vi "Machine - Add Device (SubVI).vi"(8 "error in":errorcluster, 10 "IP Address/SN":string[](array[string]), 11 "Port":string[](array[string])) -> (0 "error out":errorcluster)   [LabVIEW 2019]
uses:
  Controls/Machine - Device Type.ctl
  Controls/Sensor Setup - State.ctl
  Controls/Sensor Setup - Data Structure.ctl
  Controls/Calibration - Data Structure.ctl
  Controls/eFGV States.ctl
  Controls/Global - Data UDP.vi
panel:
  in  "Device Type":T1 items=["Unitron", "Flowtron", "Datalogger"]
  in  "Port":string
  in  "IP Address/SN List":i32(listbox)
  in  "IP Address/SN":string
  in  "Device Name":string
  in  "Status":u16(ring) items=["ACTIVE", "DISABLE"]
  in  "Close":bool
  in  "Save":bool
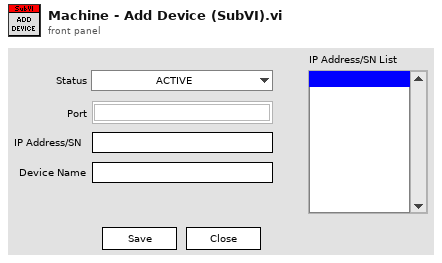
[diagram p1: front panel]
types:
  T1 = typedef "Machine - Device Type.ctl" = u16
  T2 = typedef "Sensor Setup - State.ctl" = enum16{"Init", "Idle", "Save", "Close"}
  T3 = typedef "Sensor Setup - Data Structure.ctl" = cluster{"serialno":string, "Name":string, "Channel":string, "Slope":string, "Intercept":string, "Unit":string, "Decimal":string, "New?":bool, "Data":T4, "Port":string[], "IP/SN":string[]}
  T4 = typedef "Calibration - Data Structure.ctl" = cluster{"Timeout":i32, "LC MC":dbl[], "TD MC":dbl[], "Motor Pulse":u64, "Disp M":dbl[], "LC Unit":string[], "Disp Unit":string[], "TD Unit":string[], "LC Name":string[], "TD Name":string[], "Machine":enum16{"Please Select", "Motor 1", "Motor 2", "Motor 3", "Motor 4", "Motor 5", "Motor 6", "Motor 7", "Motor 8", "Motor 9"}, "Sensor Port":enum16{"Please Select", "LC 1", "LC 2", "LC 3", "LC 4", "LC 5", "LC 6", "LC 7", "LC 8", "TD 1", "TD 2", "TD 3", "TD 4", "TD 5", "TD 6", "TD 7", "TD 8", "TD 9", "TD 10", "TD 11", "TD 12"}[]}
  T5 = typedef "eFGV States.ctl" = enum16{"Init", "Read", "Write", "Exit"}
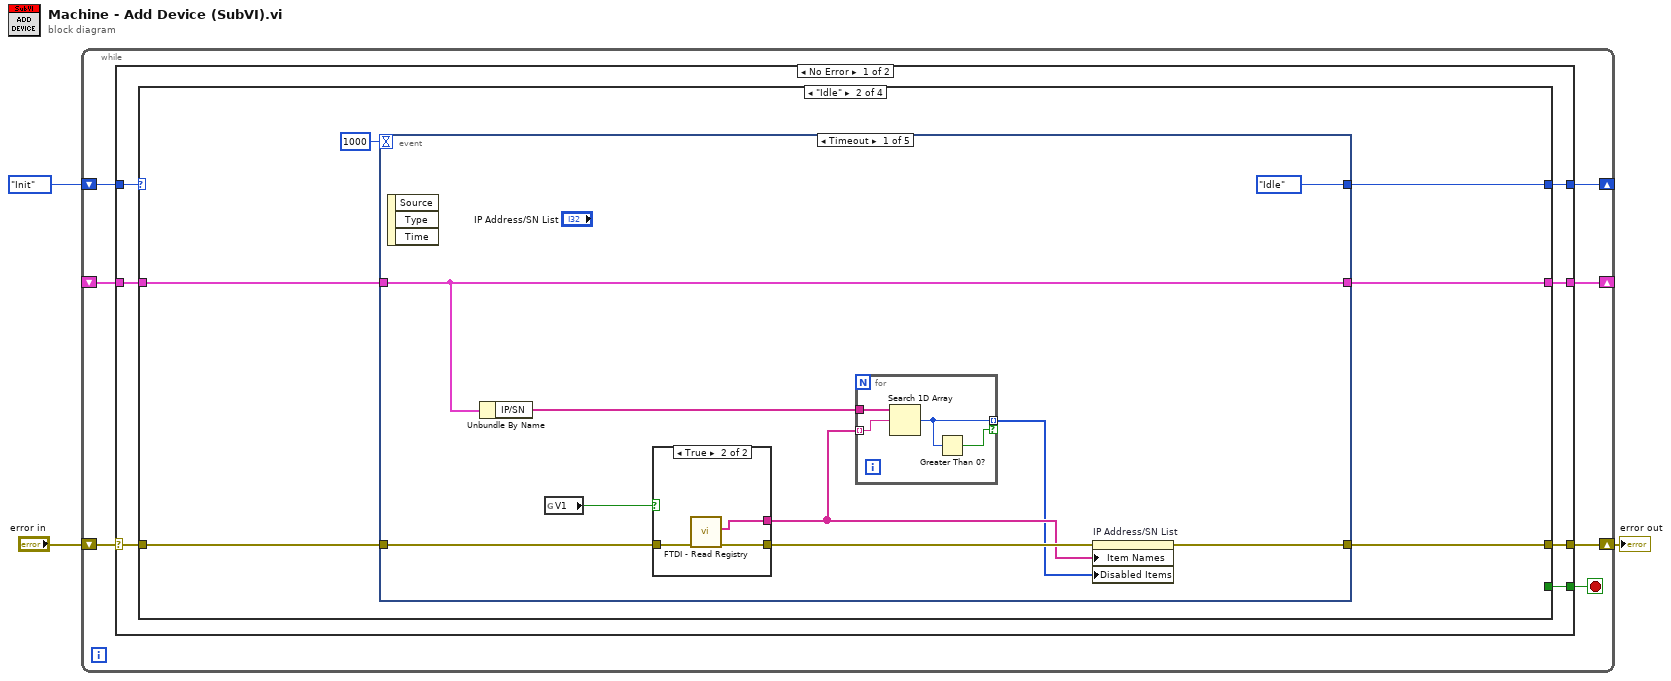
[diagram p0: block diagram]
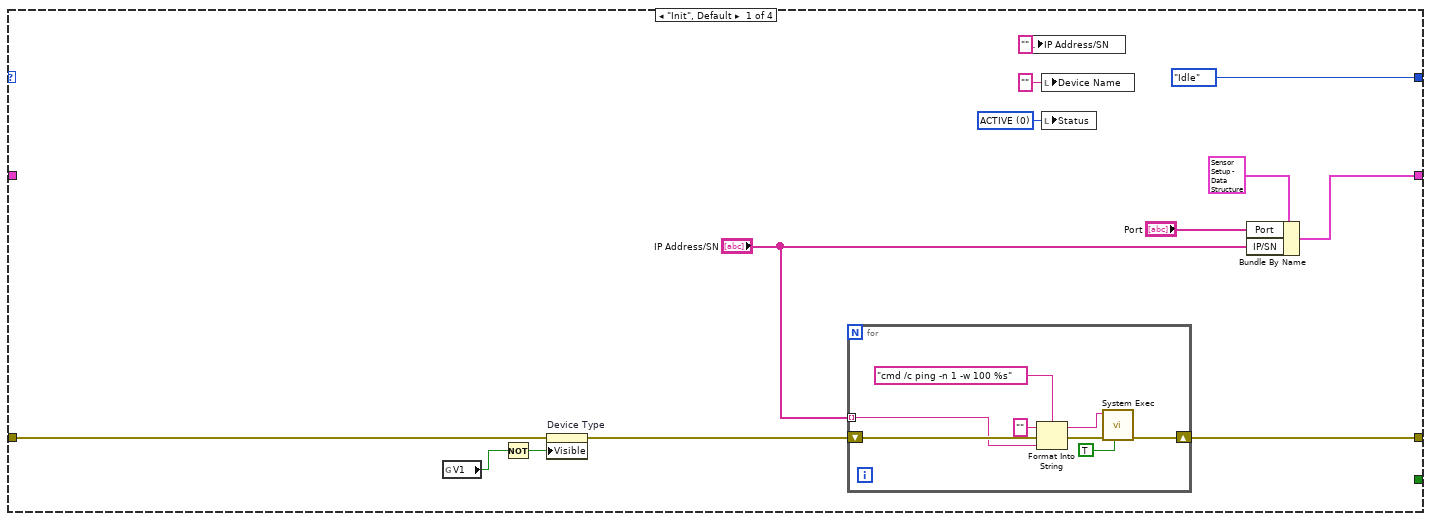
[diagram p2: hidden frame]
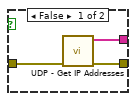
[diagram p3: hidden frame]
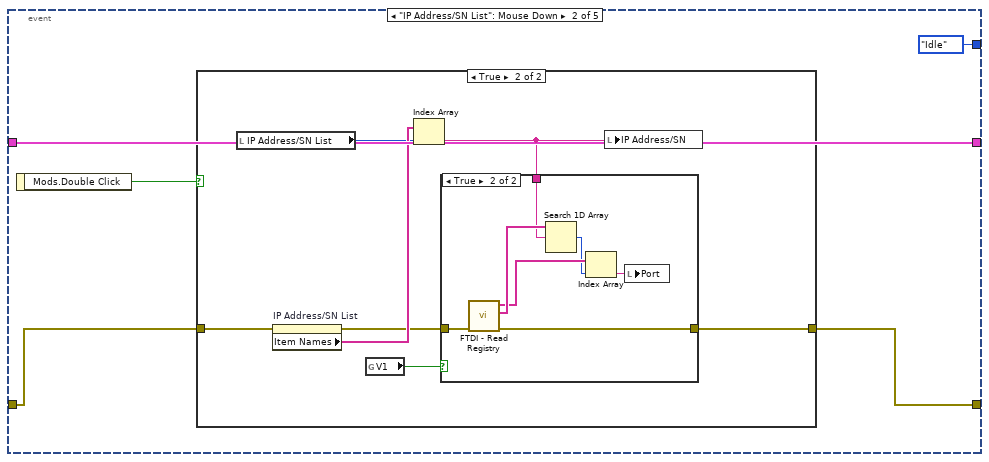
[diagram p4: hidden frame]
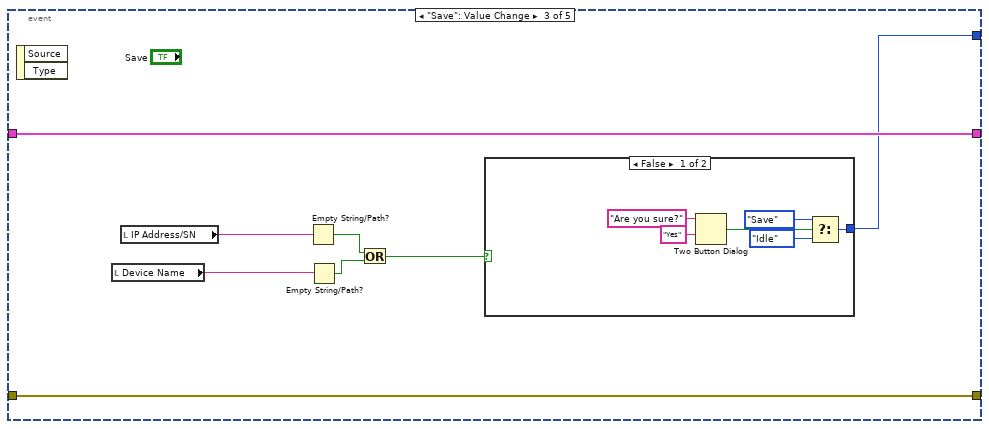
[diagram p7: hidden frame]
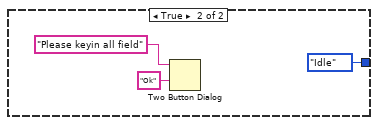
[diagram p8: hidden frame]
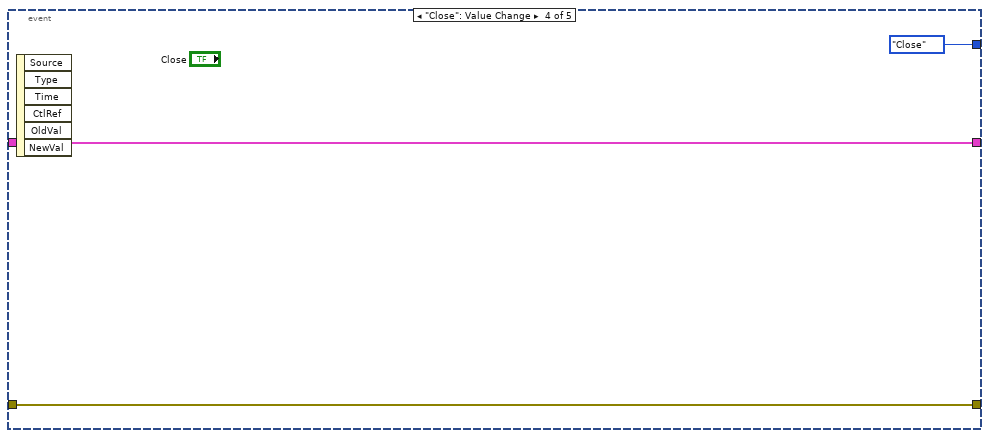
[diagram p9: hidden frame]
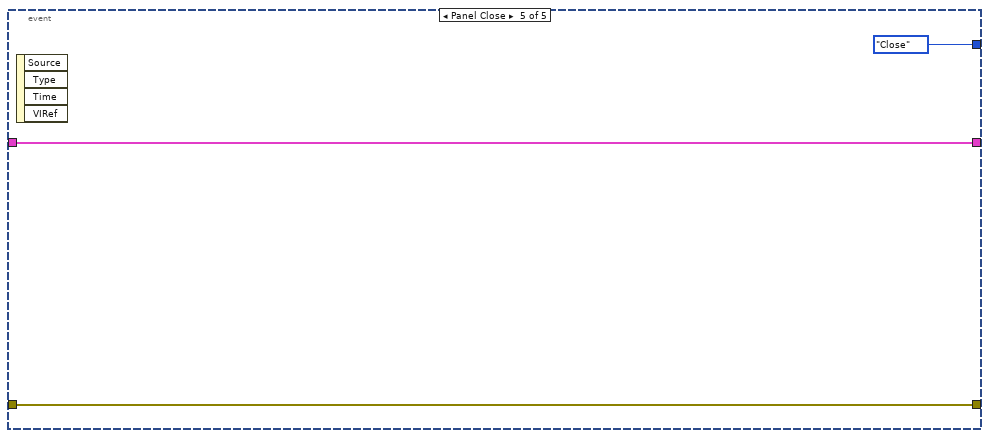
[diagram p10: hidden frame]
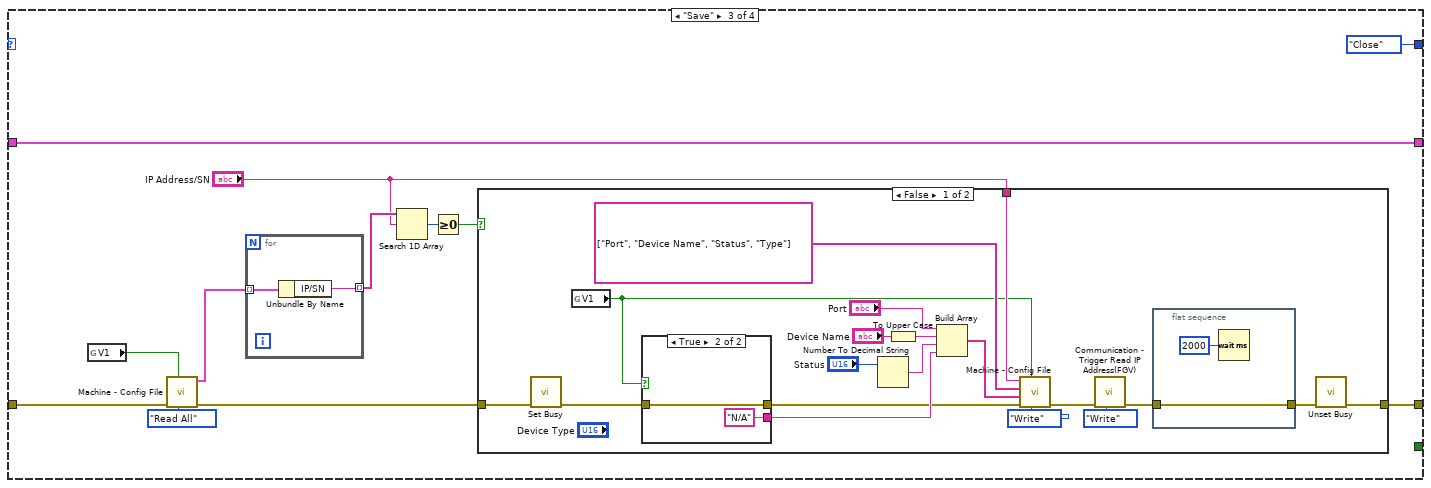
[diagram p11: hidden frame]
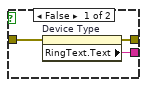
[diagram p12: hidden frame]
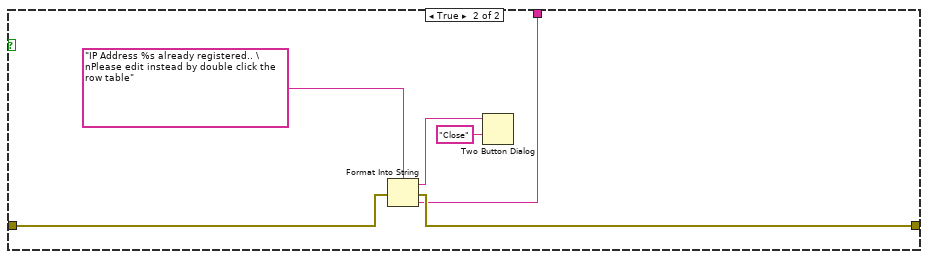
[diagram p13: hidden frame]
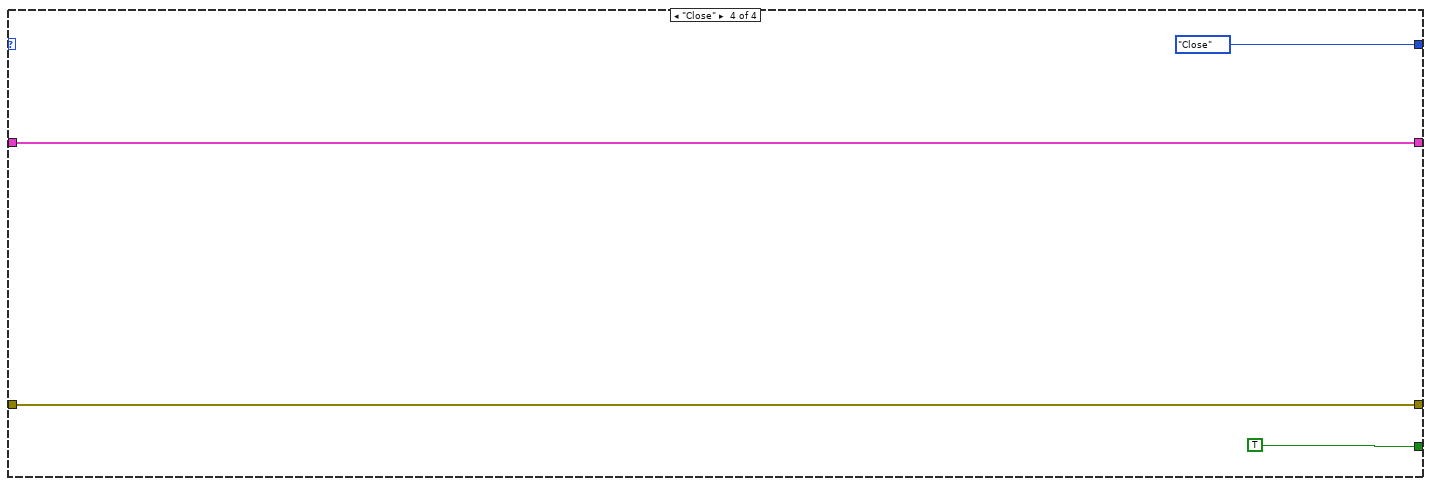
[diagram p14: hidden frame]
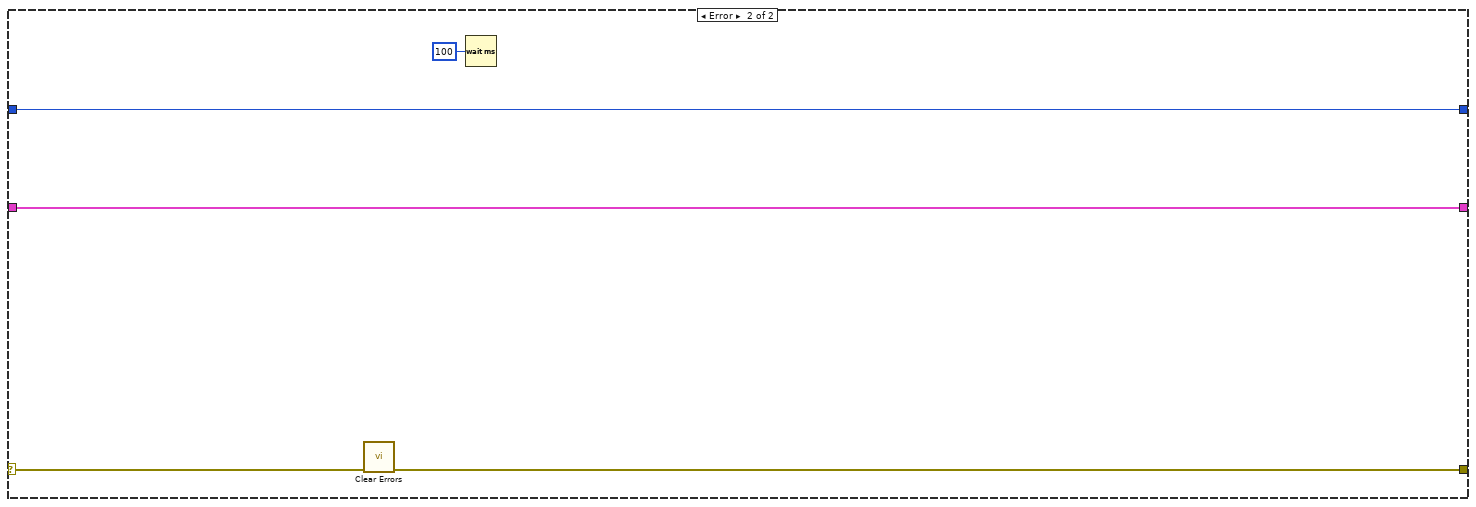
[diagram p15: hidden frame]
diagram:
  n1 = while {
    shift-right: [w9] -> _
    shift-left: Sensor_Setup_-_State."Init" -> [w10]
    shift-right: [w7] -> w1
    shift-left: "error in" -> [w8]
    shift-right: [w5] -> _
    shift-left: _ -> [w4]
    stop <- w6 stop-if-true
    n2 = case shown="No Error" w8 {
      selector: w8 -> [w14 w162]
      tunnel: w10 -> [w17 w158]
      tunnel: [w16 w158] -> w9
      tunnel: [w15 w161] -> w7
      tunnel: [w13 _] -> w6
      tunnel: [w12 w159] -> w5
      tunnel: w4 -> [w11 w159]
      frame No Error {
        n3 = case shown="\"Idle\"" w17 {
          tunnel: [Sensor_Setup_-_State."Idle" w42 Sensor_Setup_-_State."Close" Sensor_Setup_-_State."Close"] -> w16
          tunnel: [w23 w44 w118 w157] -> w15
          tunnel: w14 -> [w20 w43 w114 w157]
          tunnel: [_ _ _ TRUE] -> w13
          tunnel: [w24 w41 w117 w154] -> w12
          tunnel: w11 -> [_ w40 w117 w154]
          frame "Init", Default {
            w27 = u16 0 items=["ACTIVE", "DISABLE"] ("Status")
            n4 = global read "Global - Data UDP.vi" "V1"() -> (w19:bool)
            n5 = Not(x=w19) -> (.not. x?=w18:bool)
            n6 = property on="Device Type" class="Ring (strict)"(error in=w20, "Visible"=w18) -> (error out=w21:errorcluster)  [unwired: 1 in, 1 out]
            n7 = for {
              shift-right: [w33] -> w23
              shift-left: w21 -> [w36]
              tunnel: "IP Address/SN" -> [w32] mode=indexing
              n8 = Format Into String(format string="cmd /c ping -n 1 -w 100 %s" ("command line"), initial string="", error in=w36, w32) -> (resulting string=w31:string, error out=w37:errorcluster)
              n9 = call <vilib>:"System Exec.vi"("run minimized? (F)"=TRUE, "error in (no error)"=w37, "command line"=w31) -> ("error out"=w33:errorcluster)  [unwired: 5 in, 3 out]
            }
            n10 = local write "IP Address/SN"("" ("Serial No")) -> ()
            n11 = local write "Device Name"("" ("Device Name")) -> ()
            n12 = local write "Status"(w27) -> ()
            n13 = Bundle By Name(cluster=T3 {"serialno"="", "Name"="", "Channel"="", "Slope"="", "Intercept"="", "Unit"="", "Decimal"="", "New?"=FALSE, "Data"={"Timeout"=-1, "LC MC"=[], "TD MC"=[], "Motor Pulse"=0, "Disp M"=[], "LC Unit"=[], "Disp Unit"=[], "TD Unit"=[], "LC Name"=[], "TD Name"=[], "Machine"=enum."Please Select", "Sensor Port"=[]}, "Port"=[], "IP/SN"=[]}, "Port"="Port", "IP/SN"="IP Address/SN") -> (w24:T3)
          }
          frame "Idle" {
            n14 = event shown="[0] Timeout" {
              selector: _ -> [_ _ _ _ _]
              dyn-events: _ -> [_ _ _ _ _]
              timeout: 1000 -> [_ _ _ _ _]
              tunnel: [w52 w64 w92 w104 w107] -> w44
              tunnel: w43 -> [w51 w65 w92 w104 w107]
              tunnel: [Sensor_Setup_-_State."Idle" Sensor_Setup_-_State."Idle" w90 Sensor_Setup_-_State."Close" Sensor_Setup_-_State."Close"] -> w42
              tunnel: [w49 w68 w91 w103 w106] -> w41
              tunnel: w40 -> [w49 w68 w91 w103 w106]
              event Timeout {
                n15 = event-data() -> ()  [unwired: 1 in, 3 out]
                n16 = Unbundle By Name(w49) -> ("IP/SN"=w48:string[])
                n17 = global read "Global - Data UDP.vi" "V1"() -> (w45:bool)
                n18 = case shown="True" w45 {
                  tunnel: w51 -> [w56 w59]
                  tunnel: [w55 w58] -> w50
                  tunnel: [w54 w57] -> w47
                  frame False {
                    n19 = call "UDP - Get IP Addresses.vi"("error in"=w56) -> ("error out"=w55:errorcluster, "IP Addresses"=w54:string[])  [unwired: 9 in]
                  }
                  frame True {
                    n20 = call "FTDI - Read Registry.vi"("error in (no error)"=w59) -> ("error out"=w58:errorcluster, "Serial Number"=w57:string[])  [unwired: 8 in, 1 out]
                  }
                }
                n21 = for {
                  tunnel: w48 -> [w62]
                  tunnel: w47 -> [w63] mode=indexing
                  tunnel: [w61] -> w46 mode=indexing if=w60
                  n22 = Search 1D Array(1D array=w62, element=w63) -> (index of element=w61:i32)  [unwired: 1 in]
                  n23 = Greater Than 0?(x=w61) -> (x > 0?=w60:bool)
                }
                n24 = property on="IP Address/SN List" class="LstBox (strict)"(error in=w50, "Item Names"=w47, "Disabled Items"=w46) -> (error out=w52:errorcluster)  [unwired: 1 in, 1 out]
              }
              event "IP Address/SN List": Mouse Down {
                n25 = event-data() -> ("Mods.Double Click"=w66:bool)  [unwired: 1 in]
                n26 = case shown="True" w66 {
                  tunnel: w65 -> [w69 w76]
                  tunnel: [w69 w72] -> w64
                  frame False {
                  }
                  frame True {
                    n27 = local read "IP Address/SN List"() -> (w74:i32)
                    n28 = property on="IP Address/SN List" class="LstBox (strict)"(error in=w76) -> (error out=w73:errorcluster, "Item Names"=w75:string[])  [unwired: 1 in, 1 out]
                    n29 = global read "Global - Data UDP.vi" "V1"() -> (w70:bool)
                    n30 = Index Array(array=w75, index=w74) -> (element=w71:string)
                    n31 = case shown="True" w70 {
                      tunnel: w73 -> [w77 w84]
                      tunnel: [w77 w83] -> w72
                      tunnel: w71 -> [_ w81]
                      frame False {
                      }
                      frame True {
                        n32 = call "FTDI - Read Registry.vi"("error in (no error)"=w84) -> ("error out"=w83:errorcluster, "Serial Number"=w82:string[], "ComPort"=w80:string[])  [unwired: 8 in]
                        n33 = Search 1D Array(1D array=w82, element=w81) -> (index of element=w79:i32)  [unwired: 1 in]
                        n34 = Index Array(array=w80, index=w79) -> (element=w78:string)
                        n35 = local write "Port"(w78) -> ()
                      }
                    }
                    n36 = local write "IP Address/SN"(w71) -> ()
                  }
                }
              }
              event "Save": Value Change {
                n37 = event-data() -> ()  [unwired: 1 in, 2 out]
                n38 = local read "Device Name"() -> (w89:string)
                n39 = local read "IP Address/SN"() -> (w88:string)
                n40 = Empty String/Path?(string/path=w88) -> (empty?=w87:bool)
                n41 = Empty String/Path?(string/path=w89) -> (empty?=w86:bool)
                n42 = Or(x=w87, y=w86) -> (x .or. y?=w85:bool)
                n43 = case shown="False" w85 {
                  tunnel: [w94 Sensor_Setup_-_State."Idle" ("f")] -> w90
                  frame False {
                    n44 = Two Button Dialog(message="Are you sure?", 2:"Yes" ("T button name (\"OK\")")) -> (T button?=w96:bool)  [unwired: 1 in]
                    n45 = Select(t=Sensor_Setup_-_State."Save", s=w96, f=Sensor_Setup_-_State."Idle") -> (s? t:f=w94:T2)
                  }
                  frame True {
                    n46 = Two Button Dialog(message="Please keyin all field", 2:"Ok" ("T button name (\"OK\")")) -> ()  [unwired: 1 in, 1 out]
                  }
                }
              }
              event "Close": Value Change {
                n47 = event-data() -> ()  [unwired: 1 in, 6 out]
              }
              event Panel Close {
                n48 = event-data() -> ()  [unwired: 1 in, 4 out]
              }
            }
          }
          frame "Save" {
            n49 = global read "Global - Data UDP.vi" "V1"() -> (w108:bool)
            n50 = call "Machine - Config File.vi"("Action"=enum16{"Write", "Read", "Read All", "Remove"}."Read All", "V1"=w108, "error in (no error)"=w114) -> ("error out"=w115:errorcluster, "Value Out"=w113:cluster{"IP/SN":string, "Key Value":string[]}[])  [unwired: 7 in]
            n51 = for {
              tunnel: w113 -> [w153] mode=indexing
              tunnel: [w152] -> w112 mode=indexing
              n52 = Unbundle By Name(w153) -> ("IP/SN"=w152:string)
            }
            n53 = Search 1D Array(1D array=w112, element="IP Address/SN") -> (index of element=w110:i32)  [unwired: 1 in]
            n54 = Greater Or Equal To 0?(x=w110) -> (x >= 0?=w109:bool)
            n55 = case shown="False" w109 {
              tunnel: [w125 w150] -> w118
              tunnel: w115 -> [w127 w149]
              tunnel: "IP Address/SN" -> [w131 w147]
              frame False {
                n56 = call <vilib>:"Set Busy.vi"("error in (no error)"=w127) -> ("error out"=w123:errorcluster)  [unwired: 9 in, 1 out]
                n57 = global read "Global - Data UDP.vi" "V1"() -> (w120:bool)
                n58 = case shown="True" w120 {
                  tunnel: [w141 "N/A" ("RingText.Text")] -> w124
                  tunnel: w123 -> [w140 w143]
                  tunnel: [w139 w143] -> w122
                  frame False {
                    n59 = property on="Device Type" class="Ring (strict)"(error in=w140) -> (error out=w139:errorcluster, "RingText.Text"=w141:string)  [unwired: 1 in, 1 out]
                  }
                  frame True {
                  }
                }
                n60 = Number To Decimal String(number="Status") -> (decimal integer string=w138:string)  [unwired: 1 in]
                n61 = To Upper Case(1:"Device Name") -> (0:w132:string)
                n62 = Build Array("Port", w132, w138, w124) -> (w135:string[])
                n63 = call "Machine - Config File.vi"("Action"=enum16{"Write", "Read", "Read All", "Remove"}."Write", "V1"=w120, "error in (no error)"=w122, "Value"=w135, "Key Name"=string[] ["Port", "Device Name", "Status", "Type"], "IP/SN"=w131) -> ("error out"=w130:errorcluster)  [unwired: 4 in, 1 out]
                n64 = call "Communication - Trigger Read IP Address(FGV).vi"("Action"=eFGV_States."Write", "error in"=w130) -> ("error out"=w128:errorcluster)  [unwired: 7 in, 2 out]
                n65 = flat-sequence {
                  tunnel: [w144] -> w126
                  tunnel: w128 -> [w144]
                  frame #0 {
                    n66 = Wait (ms)(milliseconds to wait=u32 2000) -> ()  [unwired: 1 out]
                  }
                }
                n67 = call <vilib>:"Unset Busy.vi"("error in (no error)"=w126) -> ("error out"=w125:errorcluster)  [unwired: 10 in]
              }
              frame True {
                n68 = Format Into String(format string="IP Address %s already registered.. \nPlease edit instead by double click the row table" ("message"), error in=w149, w147) -> (resulting string=w146:string, error out=w150:errorcluster)  [unwired: 1 in]
                n69 = Two Button Dialog(message=w146, 2:"Close" ("T button name (\"OK\")")) -> ()  [unwired: 1 in, 1 out]
              }
            }
          }
          frame "Close" {
          }
        }
      }
      frame Error {
        n70 = call <vilib>:"Clear Errors.vi"("error in (no error)"=w162) -> ("error out"=w161:errorcluster)  [unwired: 5 in, 1 out]
        n71 = Wait (ms)(milliseconds to wait=u32 100) -> ()  [unwired: 1 out]
      }
    }
  }
  "error out" <- w1
